vi "ExampleCB.vi"(8 "error in (no error)":errorcluster, 11 "Message to LabVIEW App":T1={"Command"="zxcvbnm,", "Data"=["asdfghjk", "qwertyui"], "Script ID"=0, "LabVIEW Server ID"="zxcvbnm,", "Python Message ID"=0}) -> (0 "error out":errorcluster)   [LabVIEW 2013]
doc: "This is an example of a callback VI that you would need to write for your user application. Here we just send the message along to a queue handler. The input should be the fundamental data type, and wherever the message goes should handle it."
uses:
  LabVIEW Core/TS.lvlib
  LabVIEW Core/LabVIEW Python Connector Message.ctl
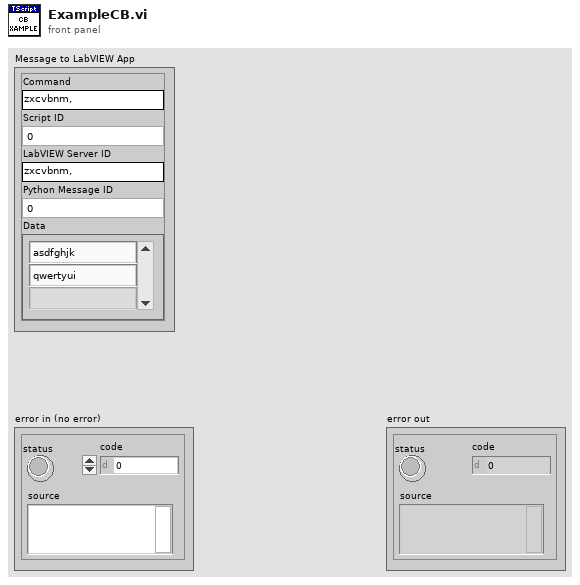
[diagram p1: front panel]
types:
  T1 = typedef "TS.lvlib/LabVIEW Python Connector Message.ctl" = cluster{"Command":string, "Data":string[], "Script ID":i64, "LabVIEW Server ID":string, "Python Message ID":i32}
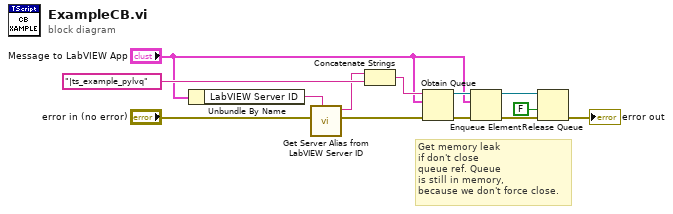
[diagram p0: block diagram]
diagram:
  # "Get memory leak\nif don't close\nqueue ref. Queue\nis still in memory,\nbecause we don't force close."
  n1 = Unbundle By Name("Message to LabVIEW App") -> ("LabVIEW Server ID"=w2:string)
  n2 = call "Get Server Alias from LabVIEW Server ID.vi"("LabVIEW Server ID"=w2, "Error In"="error in (no error)") -> ("Error Out"=w3:errorcluster, "Server Alias"=w1:string)  [unwired: 8 in]
  n3 = Concatenate Strings(w1, "|ts_example_pylvq" ("name (unnamed)")) -> (w5:string)
  n4 = Obtain Queue(name (unnamed)=w5, element data type="Message to LabVIEW App", error in (no error)=w3) -> (queue out=w10:refnum<queue>, error out=w11:errorcluster)  [unwired: 2 in, 1 out]
  n5 = Enqueue Element(queue=w10, element="Message to LabVIEW App", error in (no error)=w11) -> (queue out=w8:refnum<queue>, error out=w9:errorcluster)  [unwired: 1 in, 1 out]
  n6 = Release Queue(queue=w8, force destroy? (F)=FALSE, error in (no error)=w9) -> (error out=→"error out":errorcluster)  [unwired: 2 out]
